vi "RotateAround.vi"(8 "Target":dbl[](array[numeric]), 11 "Position":dbl[](array[numeric])) -> (4 "Output\nVelocity":dbl[](array[numeric]) format="%.2f")   [LabVIEW 2016]
uses:
  <vilib>/Analysis/coordinate.llb/Wrap Angle (scalar).vi
  <vilib>/Analysis/coordinate.llb/2D Cartesian Coordinate Rotation (Scalar).vi
  <vilib>/addons/control/pid/pid.llb/PID (DBL Array).vi
  <vilib>/addons/control/pid/NI_PID_pid.lvlib
  <vilib>/Analysis/NI_AALPro.lvlib
  <vilib>/Analysis/NI_AAL_Angle.lvlib
panel:
  in  "output range":cluster{"output high":dbl, "output low":dbl}[](array[cluster])=[{"output high"=2.0, "output low"=-2.0}] {"output low" format="%.2f"; "output high" format="%.2f"}
  in  "Reinitialize":bool
  in  "PID gains":T1(array[cluster])=[{"proportional gain (Kc)"=0.004, "integral time (Ti, min)"=0.0, "derivative time (Td, min)"=0.0}, {"proportional gain (Kc)"=1.5, "integral time (Ti, min)"=0.0, "derivative time (Td, min)"=0.0}]
  # "x centre"
  # "y centre"
  # "radius"
  # "angle around\ncentre"
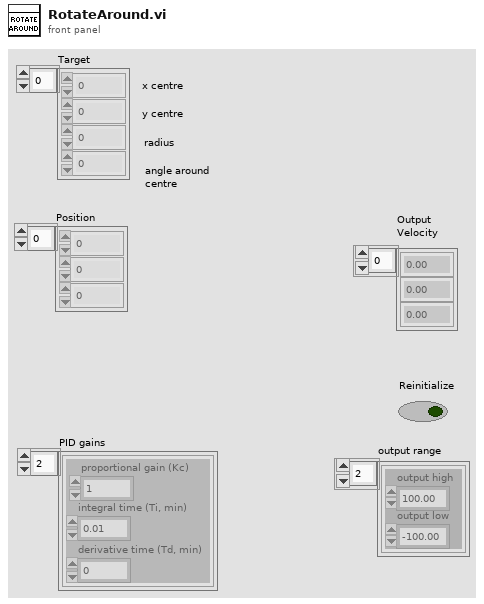
[diagram p1: front panel]
types:
  T1 = cluster{"proportional gain (Kc)":dbl, "integral time (Ti, min)":dbl, "derivative time (Td, min)":dbl}[]
  T2 = cluster{"proportional gain (Kc)":dbl, "integral time (Ti, min)":dbl, "derivative time (Td, min)":dbl}
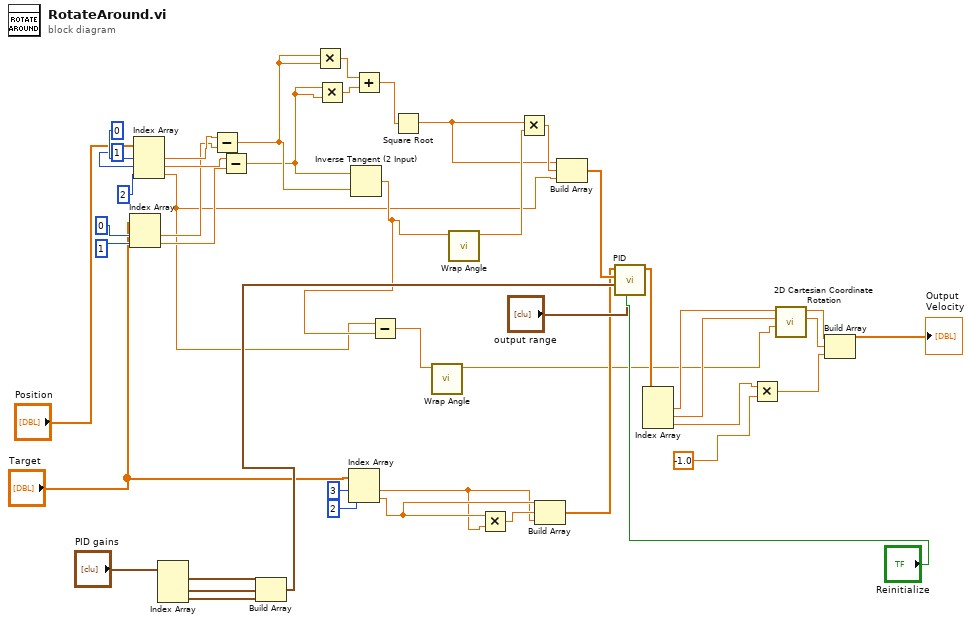
[diagram p0: block diagram]
diagram:
  n1 = Index Array(array="Target", index #1=0 ("index"), index #2=1 ("index")) -> (element #1=w5:dbl, element #2=w7:dbl)
  n2 = Index Array(array="Position", index #1=0 ("index"), index #2=1 ("index"), index #3=2 ("index")) -> (element #1=w6:dbl, element #2=w8:dbl, element #3=w1:dbl)
  n3 = Index Array(array="PID gains") -> (element #1=w39:T2, element #2=w30:T2, element #3=w31:T2)  [unwired: 3 in]
  n4 = Subtract(x=w6, y=w5) -> (x-y=w29:dbl)
  n5 = Subtract(x=w8, y=w7) -> (x-y=w28:dbl)
  n6 = Build Array(w39, w30, w31) -> (w38:T1)
  n7 = Multiply(x=w29, y=w29) -> (x*y=w33:dbl)
  n8 = Multiply(x=w28, y=w28) -> (x*y=w32:dbl)
  n9 = Index Array(array="Target", index #1=3 ("index"), index #2=2 ("index")) -> (element #1=w12:dbl, element #2=w14:dbl)
  n10 = Inverse Tangent (2 Input)(1:w29, 2:w28) -> (0:w4:dbl)
  n11 = Add(x=w33, y=w32) -> (x+y=w25:dbl)
  n12 = Subtract(x=w1, y=w4) -> (x-y=w3:dbl)
  n13 = Square Root(x=w25) -> (sqrt(x)=w15:dbl)
  n14 = call-poly <vilib>:"Wrap Angle.vi"("angle in"=w3) -> ("angle out"=w2:dbl)  [unwired: 9 in, 1 out]
  n15 = call-poly <vilib>:"Wrap Angle.vi"("angle in"=w4) -> ("angle out"=w24:dbl)  [unwired: 9 in, 1 out]
  n16 = Multiply(x=w14, y=w12) -> (x*y=w13:dbl)
  n17 = Multiply(x=w15, y=w24) -> (x*y=w18:dbl)
  n18 = Build Array(w14, w13, w12) -> (w16:dbl[])
  n19 = Build Array(w15, w18, w1) -> (w17:dbl[])
  n20 = call-poly <vilib>:"PID.vi"("reinitialize? (F)"="Reinitialize", "output range"="output range", "PID gains"=w38, "process variable"=w17, "setpoint"=w16) -> ("output"=w44:dbl[])  [unwired: 5 in, 1 out]
  n21 = Index Array(array=w44) -> (element #1=w23:dbl, element #2=w22:dbl, element #3=w10:dbl)  [unwired: 3 in]
  n22 = Multiply(x=w10, y=-1.0) -> (x*y=w9:dbl)
  n23 = call-poly <vilib>:"2D Cartesian Coordinate Rotation.vi"("theta"=w2, "y"=w22, "x"=w23) -> ("y out"=w42:dbl, "x out"=w43:dbl)  [unwired: 6 in, 1 out]
  n24 = Build Array(w43, w42, w9) -> (→"Output\nVelocity":dbl[])
